vi "SetDriveMotorOutputs.vi"(1 "RightMotorOutput":dbl, 2 "LeftMotorOutput":dbl, 4 "RightMotor1Ref":T1={"DeviceStatus"={"status"=FALSE, "code"=0, "source"=""}, "Type"=enum."PWM", "PWM"={"PWM Channel"=enum."Invalid", "DeadBand"={"Name"="", "maxPositivePwm"=0, "minPositivePwm"=0, "centerPwm"=0, "maxNegativePwm"=0, "minNegativePwm"=0, "angularRange"=0}}, "CAN"={"Device Number"=0, "Control Mode"=enum."Percent VBus", "Semaphore"=refnum, "Max Vout"=12.0, "TalonSRX Control Mode"=enum."Percent VBus"}, "Invert"=FALSE}, 6 "LeftMotor1Ref":T1={"DeviceStatus"={"status"=FALSE, "code"=0, "source"=""}, "Type"=enum."PWM", "PWM"={"PWM Channel"=enum."Invalid", "DeadBand"={"Name"="", "maxPositivePwm"=0, "minPositivePwm"=0, "centerPwm"=0, "maxNegativePwm"=0, "minNegativePwm"=0, "angularRange"=0}}, "CAN"={"Device Number"=0, "Control Mode"=enum."Percent VBus", "Semaphore"=refnum, "Max Vout"=12.0, "TalonSRX Control Mode"=enum."Percent VBus"}, "Invert"=FALSE}) -> ()   [LabVIEW 2015]
uses:
  <vilib>/Rock Robotics/WPI/MotorControl/WPI_MotorControlDeviceRef.ctl
  <vilib>/Rock Robotics/WPI/MotorControl/WPI_MotorControlType.ctl
  <vilib>/Rock Robotics/SystemInterfaces/DIO/FPGA_DIOPWMChannel.ctl
  <vilib>/Rock Robotics/WPI/PWM/WPI_PWMDeadband.ctl
  <vilib>/Rock Robotics/WPI/CAN/Jaguar/SubVIs/WPI_CANJaguar_ControlMode.ctl
  <vilib>/Rock Robotics/WPI/CAN/TalonSRX/WPI_CANTalonSRX_APIControlMode.ctl
  <vilib>/Rock Robotics/WPI/DriverStation/WPI_DriverStationRobotMode2.ctl
  Utilities/VisionGlobals.vi
panel:
  out "AutoTargetEnabled?":bool
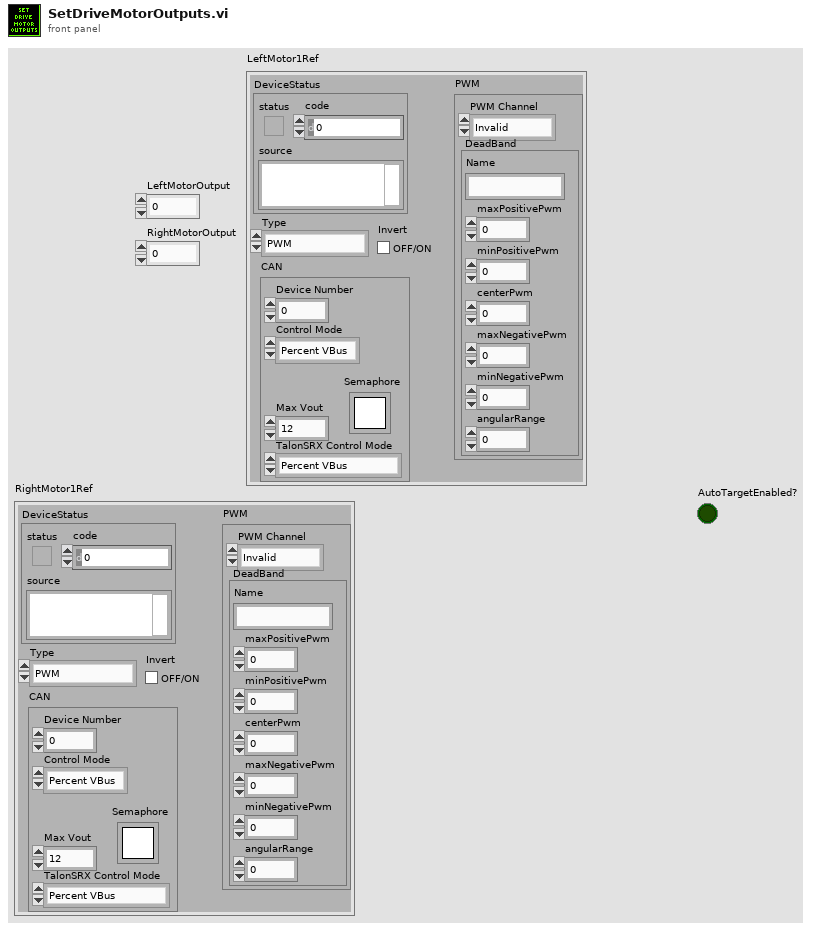
[diagram p1: front panel]
types:
  T1 = typedef "WPI_MotorControlDeviceRef.ctl" = cluster{"DeviceStatus":errorcluster, "Type":T2, "PWM":cluster{"PWM Channel":T3, "DeadBand":T4}, "CAN":cluster{"Device Number":u8, "Control Mode":T5, "Semaphore":T6, "Max Vout":dbl, "TalonSRX Control Mode":T7}, "Invert":bool}
  T2 = typedef "WPI_MotorControlType.ctl" = enum16{"PWM", "CAN", "CANTalonSRX"}
  T3 = typedef "FPGA_DIOPWMChannel.ctl" = enum8{"PWM 0", "PWM 1", "PWM 2", "PWM 3", "PWM 4", "PWM 5", "PWM 6", "PWM 7", "PWM 8", "PWM 9", "PWM MXP 0", "PWM MXP 1", "PWM MXP 2", "PWM MXP 3", "PWM MXP 4", "PWM MXP 5", "PWM MXP 6", "PWM MXP 7", "PWM MXP 8", "PWM MXP 9", "Invalid"}
  T4 = typedef "WPI_PWMDeadband.ctl" = cluster{"Name":string, "maxPositivePwm":i32, "minPositivePwm":i32, "centerPwm":i32, "maxNegativePwm":i32, "minNegativePwm":i32, "angularRange":u16}
  T5 = typedef "WPI_CANJaguar_ControlMode.ctl" = enum8{"Percent VBus", "Current", "Speed", "Position", "Voltage"}
  T6 = typedef "Semaphore RefNum" = refnum<k1>
  T7 = typedef "WPI_CANTalonSRX_APIControlMode.ctl" = enum8{"Percent VBus", "Speed", "Position", "Slave", "Unchanged / Invalid", "Voltage Compensation", "Current", "Motion Profile"}
  T8 = typedef "WPI_DriverStationRobotMode2.ctl" = enum16{"Autonomous Disabled", "Autonomous Enabled", "Teleop Disabled", "Teleop Enabled", "Disconnected", "Finish", "Test Disabled", "Test Enabled", "Emergency Stopped"}
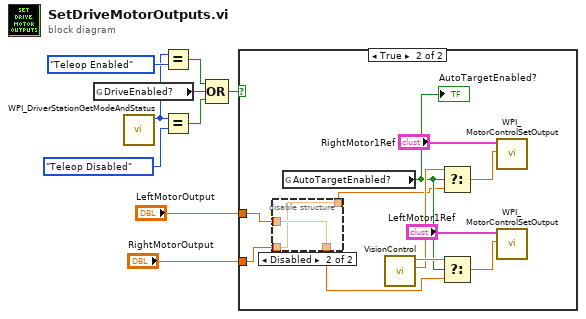
[diagram p0: block diagram]
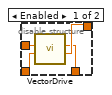
[diagram p3: hidden frame]
diagram:
  n1 = global read "VisionGlobals.vi" "DriveEnabled?"() -> (w5:bool)
  n2 = call <vilib>:"WPI_DriverStationGetModeAndStatus.vi"() -> ("Robot Mode"=w3:T8)  [unwired: 10 in, 1 out]
  n3 = Equal?(x=w3, y=WPI_DriverStationRobotMode2."Teleop Enabled") -> (x = y?=w6:bool)
  n4 = Equal?(x=w3, y=WPI_DriverStationRobotMode2."Teleop Disabled") -> (x = y?=w1:bool)
  n5 = Compound Arithmetic op=OR(w6, w5, w1) -> (w4:bool)
  n6 = case shown="True" w4 {
    tunnel: "RightMotorOutput" -> [_ w13]
    tunnel: "LeftMotorOutput" -> [_ w11]
    frame False {
    }
    frame True {
      n7 = disable-structure shown="Disabled" {
        disable-tunnel: w13 -> [w24 w25]
        disable-tunnel: [w23 w25] -> w12
        disable-tunnel: w11 -> [w22 w26]
        disable-tunnel: [w21 w26] -> w10
        frame Enabled {
          n8 = call "VectorDrive.vi"("RightMotorInput"=w24, "LeftMotorInput"=w22) -> ("RightMotorOutput"=w23:dbl, "LeftMotorOutput"=w21:dbl)  [unwired: 8 in]
        }
        frame Disabled {
        }
      }
      n9 = global read "VisionGlobals.vi" "AutoTargetEnabled?"() -> (w14:bool)
      "AutoTargetEnabled?" <- w14
      n10 = call "VisionControl.vi"() -> ("Right Drive"=w17:dbl, "Left Drive"=w18:dbl)  [unwired: 10 in]
      n11 = Select(t=w17, s=w14, f=w12) -> (s? t:f=w16:dbl)
      n12 = Select(t=w18, s=w14, f=w10) -> (s? t:f=w15:dbl)
      n13 = call <vilib>:"WPI_MotorControlSetOutput.vi"("Output"=w16, "MotorControlDevRef"="RightMotor1Ref") -> ()  [unwired: 7 in, 3 out]
      n14 = call <vilib>:"WPI_MotorControlSetOutput.vi"("Output"=w15, "MotorControlDevRef"="LeftMotor1Ref") -> ()  [unwired: 7 in, 3 out]
    }
  }
